vi "Check Motor Busy.vi"(8 "error in (no error)":errorcluster, 11 "VISA resource name":refnum<visa-resource-name>) -> (0 "error out":errorcluster, 2 "busy?":bool, 3 "VISA resource name out":refnum<visa-resource-name>)   [LabVIEW 2009, in "JY-SPEX-TRIAX.lvlib"]
doc: "Used to poll the spectrometer after motor move or slit move commands are issued in order to see if the spectrometer is done moving."
uses:
  JY-SPEX-TRIAX.lvlib
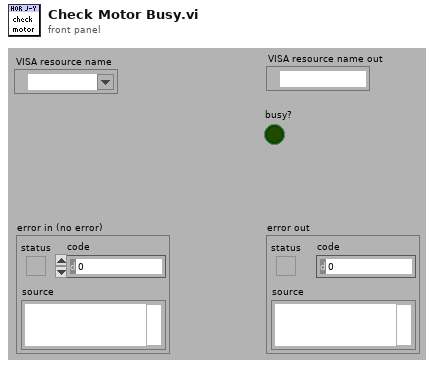
[diagram p1: front panel]
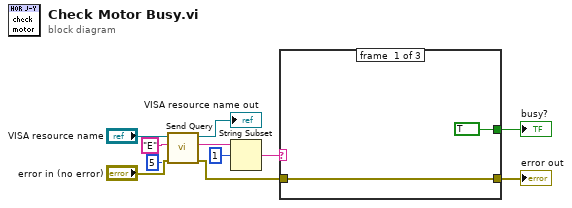
[diagram p0: block diagram]
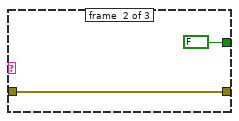
[diagram p2: hidden frame]
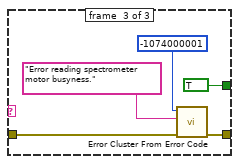
[diagram p3: hidden frame]
diagram:
  n1 = call "Send Query.vi"("error in (no error)"="error in (no error)", "byte count"=u32 5, "write buffer"="E", "VISA resource name"="VISA resource name") -> ("error out"=w4:errorcluster, "read buffer"=w7:string, "VISA resource name out"=→"VISA resource name out":refnum<visa-resource-name>)  [unwired: 5 out]
  n2 = String Subset(string=w7, offset (0)=1) -> (substring=w5:string)  [unwired: 1 out]
  n3 = case shown="Default" w5 {
    tunnel: w4 -> [w13 w15 w17]
    tunnel: [w13 w15 w18] -> w2
    tunnel: [TRUE FALSE TRUE] -> w1
    frame #0 {
    }
    frame #1 {
    }
    frame #2 {
      n4 = call <vilib>:"Error Cluster From Error Code.vi"("error in (no error)"=w17, "error message (\"\")"="Error reading spectrometer motor busyness." ("error message (\"\")"), "error code (0)"=-1074000001) -> ("error out"=w18:errorcluster)  [unwired: 1 in, 5 out]
    }
  }
  "busy?" <- w1
  "error out" <- w2
